vi "GetPathInfo.vi"(10 "End Point":T2, 11 "Start Point":T2) -> (0 "Elevator Command":T1, 2 "Theta Final":dbl, 3 "Points":cluster{"X Points":dbl[], "Y Points":dbl[]})   [LabVIEW 2017]
uses:
  KeyPoints.ctl
  CommandTypes/LiftCommands.ctl
  KeyPointInfo.ctl
  <userlib>/836-Library/System/QCP_V2/QCPSupportCode/QCPData.ctl
  <userlib>/836-Library/System/QCP_V2/QCPSupportCode/QCP_GetDbl.vi
panel:
  out "Finnish Angle":dbl
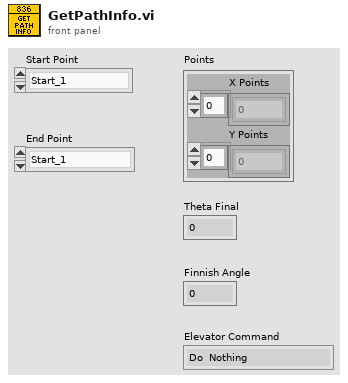
[diagram p1: front panel]
types:
  T1 = typedef "LiftCommands.ctl" = enum16{"Do  Nothing", "Manuel", "Home", "Ground", "To Switch", "To Scale Low", "To Scale Medium", "To Scale High"}
  T2 = typedef "KeyPoints.ctl" = enum16{"Start_1", "Start_2", "Start_3", "Switch_L", "Switch_R", "Scale_L", "Scale_R", "Cube_1", "Cube_2", "Cube_3", "Cube_4", "Cube_5", "Cube_6", "CubeAcq_L", "CubeAcq_R", "Switch_Back_L", "Switch_Back_R"}
  T3 = typedef "KeyPointInfo.ctl" = cluster{"Point Name":T2, "Angle At Point":dbl, "Elevator Command":T1}
  T4 = typedef "Semaphore RefNum" = refnum<k1>
  T5 = cluster{"Data Value Refnum":refnum<data-value>, "semaphore":T4}
  T6 = enum16{"[0, 360]", "[-180, 180]", "[0, 2PI]", "[-PI, PI]"}
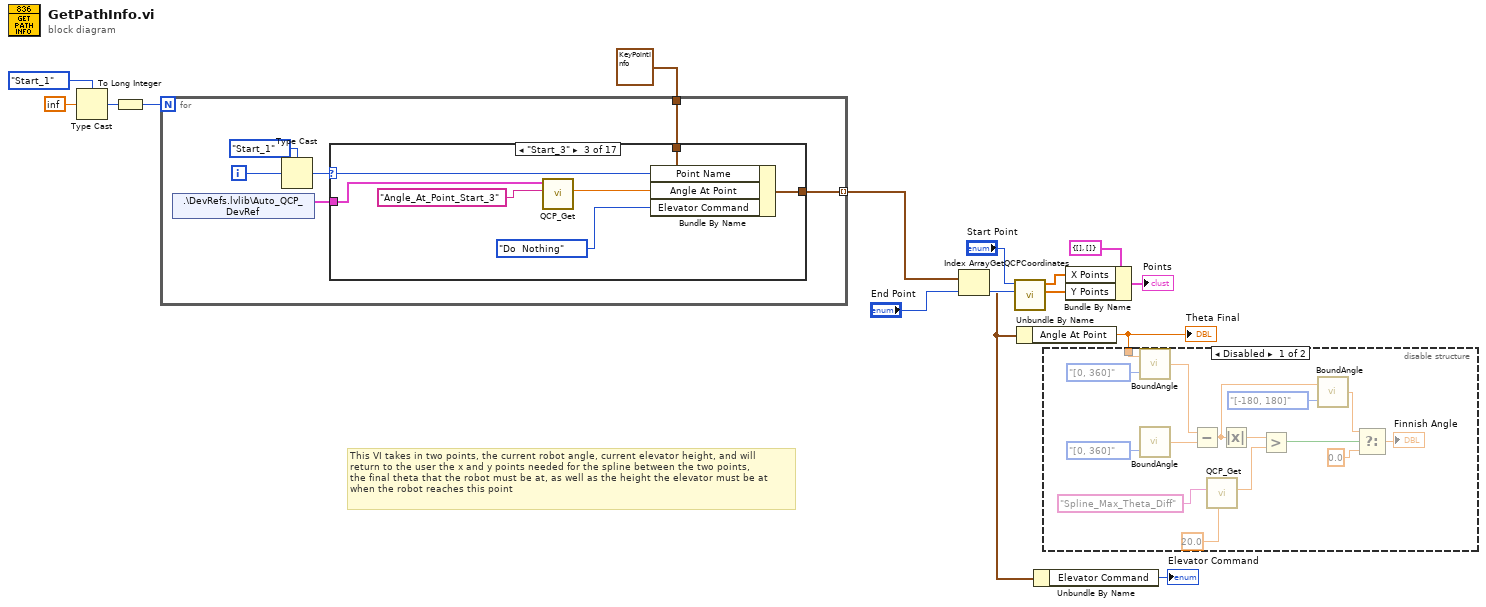
[diagram p0: block diagram]
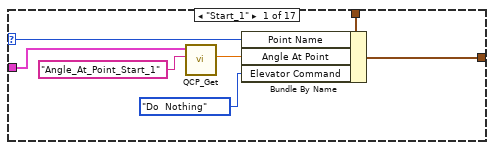
[diagram p3: hidden frame]
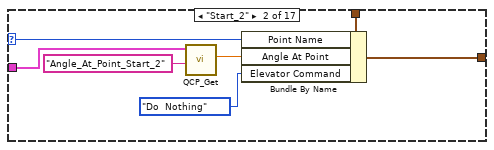
[diagram p4: hidden frame]
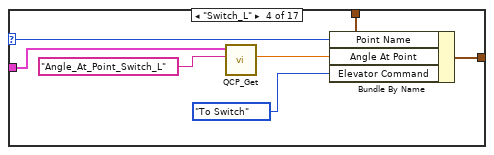
[diagram p5: hidden frame]
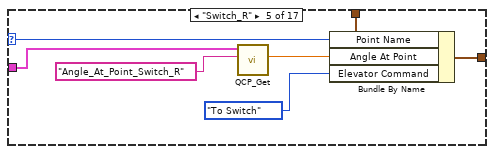
[diagram p6: hidden frame]
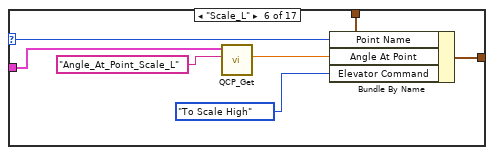
[diagram p7: hidden frame]
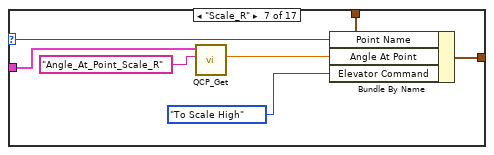
[diagram p8: hidden frame]
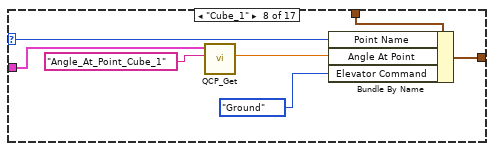
[diagram p9: hidden frame]
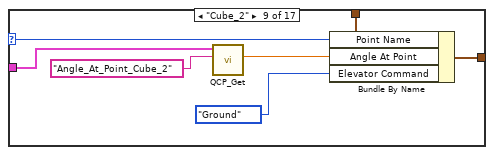
[diagram p10: hidden frame]
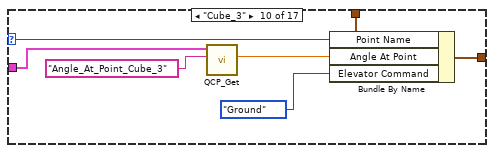
[diagram p11: hidden frame]
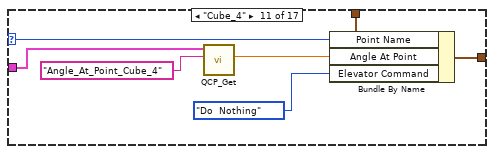
[diagram p12: hidden frame]
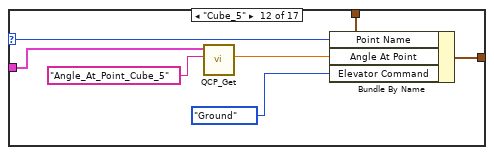
[diagram p13: hidden frame]
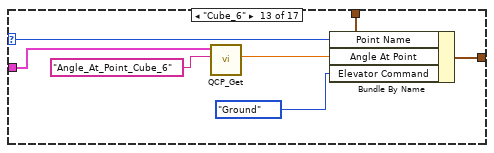
[diagram p14: hidden frame]
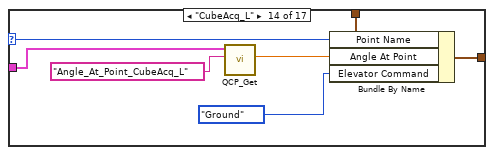
[diagram p15: hidden frame]
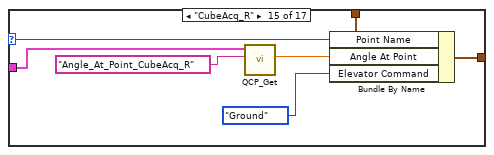
[diagram p16: hidden frame]
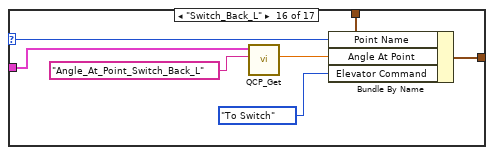
[diagram p17: hidden frame]
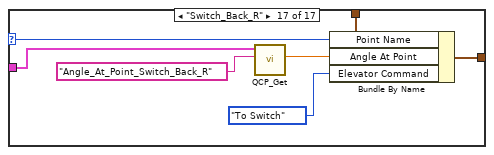
[diagram p18: hidden frame]
diagram:
  # "This VI takes in two points, the current robot angle, current elevator height, and will\nreturn to the user the x and y points needed for the spline between the two points,\nthe final theta that the robot must be at, as well as the height the elevator must be at\nwhen the robot reaches this point"
  n1 = Type Cast(type=KeyPoints."Start_1" ("Start Point"), x=inf) -> (*(type *) &x=w12:T2)
  n2 = To Long Integer(number=w12) -> (32bit integer=w13:i32)
  n3 = for {
    N: w13 -> [_]
    tunnel: T3 {"Point Name"=enum."Start_1", "Angle At Point"=0.0, "Elevator Command"=enum."Do  Nothing"} -> [w18]
    tunnel: [w17] -> w10 mode=indexing
    i -> [w21]
    n4 = shared-variable ".\\DevRefs.lvlib\\Auto_QCP_DevRef"() -> (w16:T5)  [unwired: 1 in, 1 out]
    n5 = Type Cast(type=KeyPoints."Start_1" ("Start Point"), x=w21) -> (*(type *) &x=w19:T2)
    n6 = case shown="\"Start_3\"" w19 {
      selector: w19 -> [w27 w34 w41 w48 w55 w62 w70 w76 w83 w90 w97 w104 w111 w118 w125 w132 w139]
      tunnel: w18 -> [w28 w35 w42 w49 w56 w63 w66 w77 w84 w91 w98 w105 w112 w119 w126 w133 w140]
      tunnel: [w26 w33 w40 w47 w54 w61 w69 w75 w82 w89 w96 w103 w110 w117 w124 w131 w138] -> w17
      tunnel: w16 -> [w23 w31 w38 w45 w52 w59 w67 w73 w80 w87 w94 w101 w108 w115 w122 w129 w136]
      frame "Start_1" {
        n7 = call-poly <userlib>:"QCP_Get.vi"("Value Name"="Angle_At_Point_Start_1", "QCP_DevRef_In"=w23) -> ("Value"=w24:dbl)  [unwired: 7 in, 2 out]
        n8 = Bundle By Name(cluster=w28, "Point Name"=w27, "Angle At Point"=w24, "Elevator Command"=LiftCommands."Do  Nothing") -> (w26:T3)
      }
      frame "Start_2" {
        n9 = call-poly <userlib>:"QCP_Get.vi"("Value Name"="Angle_At_Point_Start_2", "QCP_DevRef_In"=w31) -> ("Value"=w30:dbl)  [unwired: 7 in, 2 out]
        n10 = Bundle By Name(cluster=w35, "Point Name"=w34, "Angle At Point"=w30, "Elevator Command"=LiftCommands."Do  Nothing") -> (w33:T3)
      }
      frame "Start_3" {
        n11 = call-poly <userlib>:"QCP_Get.vi"("Value Name"="Angle_At_Point_Start_3", "QCP_DevRef_In"=w38) -> ("Value"=w37:dbl)  [unwired: 7 in, 2 out]
        n12 = Bundle By Name(cluster=w42, "Point Name"=w41, "Angle At Point"=w37, "Elevator Command"=LiftCommands."Do  Nothing") -> (w40:T3)
      }
      frame "Switch_L" {
        n13 = call-poly <userlib>:"QCP_Get.vi"("Value Name"="Angle_At_Point_Switch_L", "QCP_DevRef_In"=w45) -> ("Value"=w44:dbl)  [unwired: 7 in, 2 out]
        n14 = Bundle By Name(cluster=w49, "Point Name"=w48, "Angle At Point"=w44, "Elevator Command"=LiftCommands."To Switch") -> (w47:T3)
      }
      frame "Switch_R" {
        n15 = call-poly <userlib>:"QCP_Get.vi"("Value Name"="Angle_At_Point_Switch_R", "QCP_DevRef_In"=w52) -> ("Value"=w51:dbl)  [unwired: 7 in, 2 out]
        n16 = Bundle By Name(cluster=w56, "Point Name"=w55, "Angle At Point"=w51, "Elevator Command"=LiftCommands."To Switch") -> (w54:T3)
      }
      frame "Scale_L" {
        n17 = call-poly <userlib>:"QCP_Get.vi"("Value Name"="Angle_At_Point_Scale_L", "QCP_DevRef_In"=w59) -> ("Value"=w58:dbl)  [unwired: 7 in, 2 out]
        n18 = Bundle By Name(cluster=w63, "Point Name"=w62, "Angle At Point"=w58, "Elevator Command"=LiftCommands."To Scale High") -> (w61:T3)
      }
      frame "Scale_R" {
        n19 = call-poly <userlib>:"QCP_Get.vi"("Value Name"="Angle_At_Point_Scale_R", "QCP_DevRef_In"=w67) -> ("Value"=w65:dbl)  [unwired: 7 in, 2 out]
        n20 = Bundle By Name(cluster=w66, "Point Name"=w70, "Angle At Point"=w65, "Elevator Command"=LiftCommands."To Scale High") -> (w69:T3)
      }
      frame "Cube_1" {
        n21 = call-poly <userlib>:"QCP_Get.vi"("Value Name"="Angle_At_Point_Cube_1", "QCP_DevRef_In"=w73) -> ("Value"=w72:dbl)  [unwired: 7 in, 2 out]
        n22 = Bundle By Name(cluster=w77, "Point Name"=w76, "Angle At Point"=w72, "Elevator Command"=LiftCommands."Ground") -> (w75:T3)
      }
      frame "Cube_2" {
        n23 = call-poly <userlib>:"QCP_Get.vi"("Value Name"="Angle_At_Point_Cube_2", "QCP_DevRef_In"=w80) -> ("Value"=w79:dbl)  [unwired: 7 in, 2 out]
        n24 = Bundle By Name(cluster=w84, "Point Name"=w83, "Angle At Point"=w79, "Elevator Command"=LiftCommands."Ground") -> (w82:T3)
      }
      frame "Cube_3" {
        n25 = call-poly <userlib>:"QCP_Get.vi"("Value Name"="Angle_At_Point_Cube_3", "QCP_DevRef_In"=w87) -> ("Value"=w86:dbl)  [unwired: 7 in, 2 out]
        n26 = Bundle By Name(cluster=w91, "Point Name"=w90, "Angle At Point"=w86, "Elevator Command"=LiftCommands."Ground") -> (w89:T3)
      }
      frame "Cube_4" {
        n27 = call-poly <userlib>:"QCP_Get.vi"("Value Name"="Angle_At_Point_Cube_4", "QCP_DevRef_In"=w94) -> ("Value"=w93:dbl)  [unwired: 7 in, 2 out]
        n28 = Bundle By Name(cluster=w98, "Point Name"=w97, "Angle At Point"=w93, "Elevator Command"=LiftCommands."Do  Nothing") -> (w96:T3)
      }
      frame "Cube_5" {
        n29 = call-poly <userlib>:"QCP_Get.vi"("Value Name"="Angle_At_Point_Cube_5", "QCP_DevRef_In"=w101) -> ("Value"=w100:dbl)  [unwired: 7 in, 2 out]
        n30 = Bundle By Name(cluster=w105, "Point Name"=w104, "Angle At Point"=w100, "Elevator Command"=LiftCommands."Ground") -> (w103:T3)
      }
      frame "Cube_6" {
        n31 = call-poly <userlib>:"QCP_Get.vi"("Value Name"="Angle_At_Point_Cube_6", "QCP_DevRef_In"=w108) -> ("Value"=w107:dbl)  [unwired: 7 in, 2 out]
        n32 = Bundle By Name(cluster=w112, "Point Name"=w111, "Angle At Point"=w107, "Elevator Command"=LiftCommands."Ground") -> (w110:T3)
      }
      frame "CubeAcq_L" {
        n33 = call-poly <userlib>:"QCP_Get.vi"("Value Name"="Angle_At_Point_CubeAcq_L", "QCP_DevRef_In"=w115) -> ("Value"=w114:dbl)  [unwired: 7 in, 2 out]
        n34 = Bundle By Name(cluster=w119, "Point Name"=w118, "Angle At Point"=w114, "Elevator Command"=LiftCommands."Ground") -> (w117:T3)
      }
      frame "CubeAcq_R" {
        n35 = call-poly <userlib>:"QCP_Get.vi"("Value Name"="Angle_At_Point_CubeAcq_R", "QCP_DevRef_In"=w122) -> ("Value"=w121:dbl)  [unwired: 7 in, 2 out]
        n36 = Bundle By Name(cluster=w126, "Point Name"=w125, "Angle At Point"=w121, "Elevator Command"=LiftCommands."Ground") -> (w124:T3)
      }
      frame "Switch_Back_L" {
        n37 = call-poly <userlib>:"QCP_Get.vi"("Value Name"="Angle_At_Point_Switch_Back_L", "QCP_DevRef_In"=w129) -> ("Value"=w128:dbl)  [unwired: 7 in, 2 out]
        n38 = Bundle By Name(cluster=w133, "Point Name"=w132, "Angle At Point"=w128, "Elevator Command"=LiftCommands."To Switch") -> (w131:T3)
      }
      frame "Switch_Back_R" {
        n39 = call-poly <userlib>:"QCP_Get.vi"("Value Name"="Angle_At_Point_Switch_Back_R", "QCP_DevRef_In"=w136) -> ("Value"=w135:dbl)  [unwired: 7 in, 2 out]
        n40 = Bundle By Name(cluster=w140, "Point Name"=w139, "Angle At Point"=w135, "Elevator Command"=LiftCommands."To Switch") -> (w138:T3)
      }
    }
  }
  n41 = Index Array(array=w10, index="End Point") -> (element=w2:T3)
  n42 = call "GetQCPCoordinates.vi"("Stop Point"="End Point", "Start Point"="Start Point") -> ("X coordinates"=w4:dbl[], "Y coodinates"=w5:dbl[])  [unwired: 8 in]
  n43 = Unbundle By Name(w2) -> ("Angle At Point"=w9:dbl)
  "Theta Final" <- w9
  n44 = Unbundle By Name(w2) -> ("Elevator Command"=→"Elevator Command":T1)
  n45 = disable-structure shown="Disabled" {
    disable-tunnel: w9 -> [w142 _]
    frame Disabled {
      n46 = call <userlib>:"BoundAngle.vi"("Type"=T6."[0, 360]", "Angle"=w142) -> ("Bound Angle"=w141:dbl)
      n47 = call <userlib>:"BoundAngle.vi"("Type"=T6."[0, 360]") -> ("Bound Angle"=w144:dbl)  [unwired: 1 in]
      n48 = Subtract(x=w141, y=w144) -> (x-y=w148:dbl)
      n49 = call-poly <userlib>:"QCP_Get.vi"("Default Value"=20.0, "Value Name"="Spline_Max_Theta_Diff") -> ("Value"=w153:dbl)  [unwired: 7 in, 2 out]
      n50 = Absolute Value(x=w148) -> (abs(x)=w150:dbl)
      n51 = Greater?(x=w150, y=w153) -> (0:w152:bool)
      n52 = call <userlib>:"BoundAngle.vi"("Type"=T6."[-180, 180]", "Angle"=w148) -> ("Bound Angle"=w147:dbl)
      n53 = Select(t=w147, s=w152, f=0.0) -> (s? t:f=→"Finnish Angle":dbl)
    }
    frame Enabled {
    }
  }
  n54 = Bundle By Name(cluster=cluster{"X Points":dbl[], "Y Points":dbl[]} {"X Points"=[], "Y Points"=[]} ("Points"), "X Points"=w5, "Y Points"=w4) -> (→"Points":cluster{"X Points":dbl[], "Y Points":dbl[]})
